vi "Conversão parametros PRBS.vi"(1 "Seed bomba 2":i32, 2 "Seed bomba 1":i32, 3 "Duração da excitação (s)":i32, 4 "Periodo":i32) -> (0 "PRBS Parameters":T1(array[cluster]) {"polynomial order" max=512; "seed" format="%.0x"})   [LabVIEW 2015]
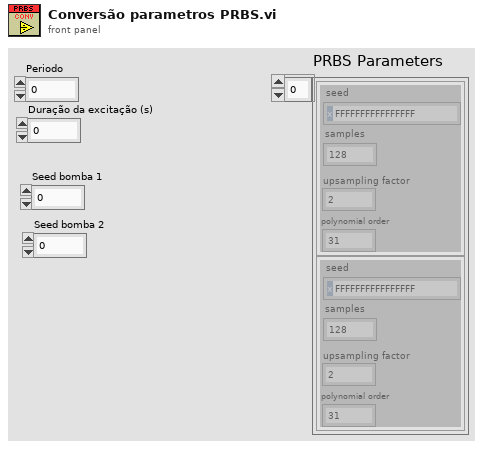
[diagram p1: front panel]
types:
  T1 = cluster{"seed":i64, "samples":i64, "upsampling factor":i32, "polynomial order":i32}[]
  T2 = cluster{"seed":i64, "samples":i64, "upsampling factor":i32, "polynomial order":i32}
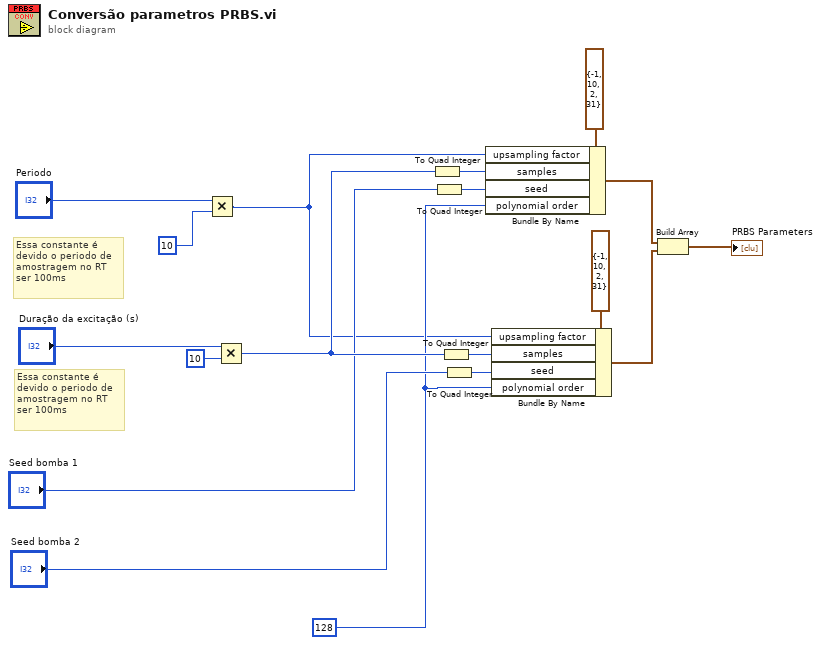
[diagram p0: block diagram]
diagram:
  w4 = 128
  # "Essa constante é\ndevido o periodo de\namostragem no RT\nser 100ms"
  # "Essa constante é\ndevido o periodo de\namostragem no RT\nser 100ms"
  n1 = Multiply(x="Periodo", y=10) -> (x*y=w1:i32)
  n2 = Multiply(x="Duração da excitação (s)", y=10) -> (x*y=w13:i32)
  n3 = To Quad Integer(1:w13) -> (0:w14:i64)
  n4 = To Quad Integer(1:"Seed bomba 1") -> (0:w10:i64)
  n5 = To Quad Integer(1:w13) -> (0:w9:i64)
  n6 = To Quad Integer(1:"Seed bomba 2") -> (0:w8:i64)
  n7 = Bundle By Name(cluster=T2 {"seed"=-1, "samples"=10, "upsampling factor"=2, "polynomial order"=31} ("Cluster"), "upsampling factor"=w1, "samples"=w14, "seed"=w10, "polynomial order"=w4) -> (w7:T2)
  n8 = Bundle By Name(cluster=T2 {"seed"=-1, "samples"=10, "upsampling factor"=2, "polynomial order"=31} ("Cluster"), "upsampling factor"=w1, "samples"=w9, "seed"=w8, "polynomial order"=w4) -> (w6:T2)
  n9 = Build Array(w7, w6) -> (→"PRBS Parameters":T1)
